vi "Y5140_RdCurr.vi"(8 "error in (no error)":errorcluster caption="错误输入（无错误）", 11 "MyIndex":u8) -> (0 "error out":errorcluster caption="错误输出", 1 "T/F":bool, 2 "Value":sgl)   [LabVIEW 2015]
uses:
  <vilib>/Instr/_visa.llb/VISA Configure Serial Port (Instr).vi
panel:
  out "VISA":refnum<visa-resource-name> caption="VISA资源名称输出"
  out "Rx":string
  out "Tx":string
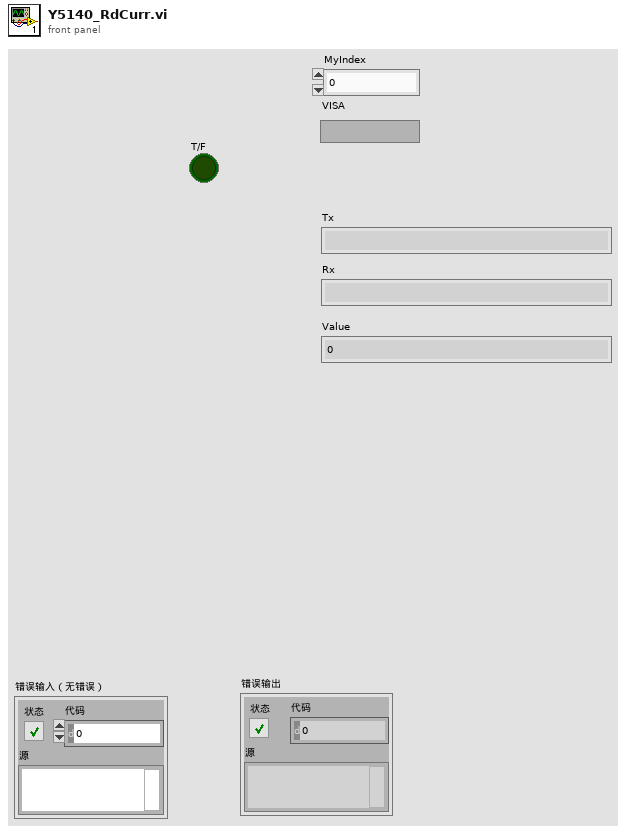
[diagram p1: front panel]
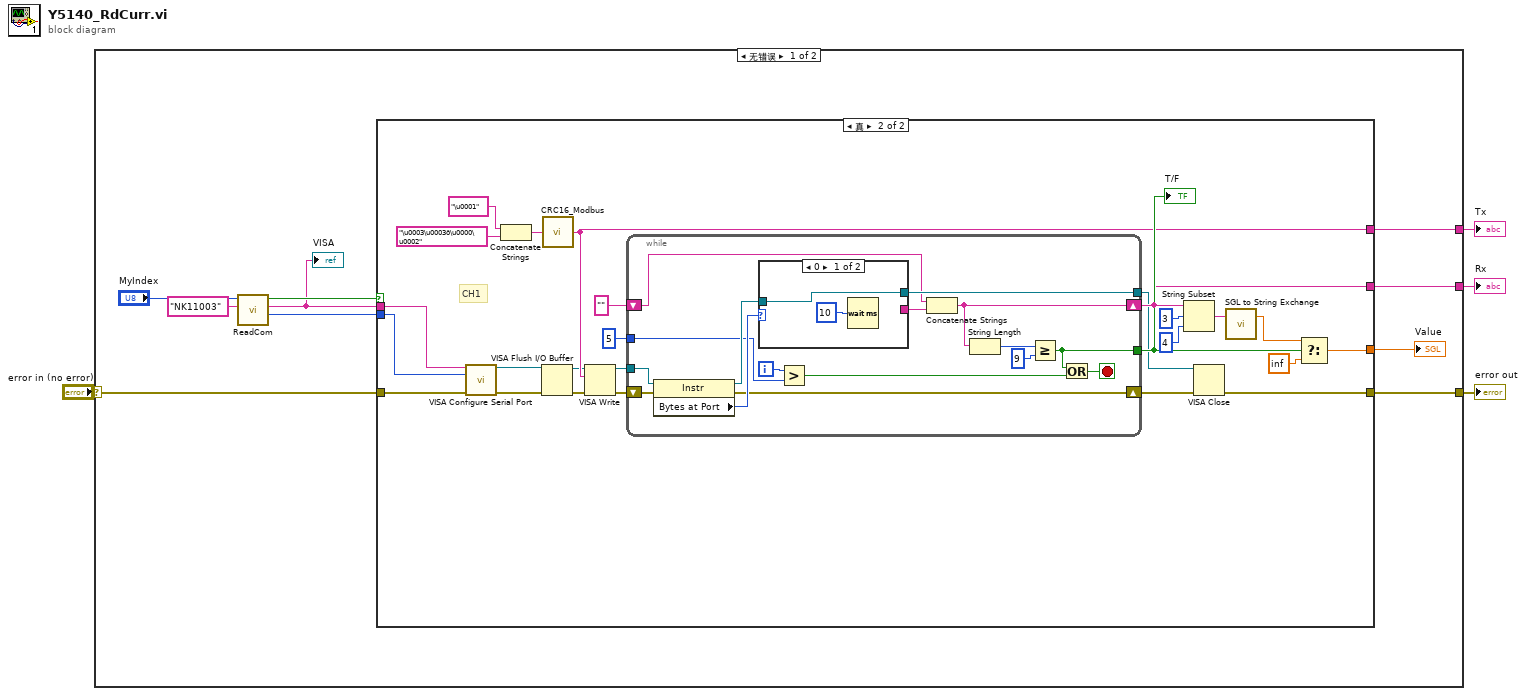
[diagram p0: block diagram]
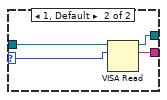
[diagram p3: hidden frame]
diagram:
  n1 = case shown="无错误" "error in (no error)" {
    selector: "error in (no error)" -> [w13 w63]
    tunnel: [w12 w63] -> w3
    tunnel: [w11 _] -> w2
    tunnel: [w10 _] -> w1
    frame No Error {
      n2 = call "ReadCom.vi"("仪器名称"="NK11003", "MyIndex"="MyIndex") -> ("Baudrate"=w5:i32, "COM"=w6:string, "OK?"=w7:bool)  [unwired: 7 in]
      "VISA" <- w6
      n3 = case shown="真" w7 {
        tunnel: [_ w39] -> w14
        tunnel: w13 -> [_ w38]
        tunnel: [_ w16] -> w12
        tunnel: [_ w36] -> w11
        tunnel: [_ w35] -> w10
        tunnel: w6 -> [_ w18]
        tunnel: w5 -> [_ w19]
        frame False {
        }
        frame True {
          # "CH1"
          n4 = call-poly "VISA Configure Serial Port"("VISA resource name"=w18, "baud rate (9600)"=w19, "error in (no error)"=w38) -> ("VISA resource name out"=w17:refnum<visa-resource-name>, "error out"=w20:errorcluster)  [unwired: 11 in]
          n5 = Concatenate Strings("\u0001", "\u0003\u0003ð\u0000\u0002") -> (w22:string)
          n6 = VISA Flush I/O Buffer(VISA resource name=w17, error in (no error)=w20) -> (VISA resource name out=w34:refnum<visa-resource-name>, error out=w33:errorcluster)  [unwired: 1 in]
          n7 = call "CRC16_Modbus.vi"("需要校验的数据"=w22) -> ("String+CRC16"=w36:string)
          n8 = VISA Write(VISA resource name=w34, write buffer=w36, error in (no error)=w33) -> (VISA resource name out=w32:refnum<visa-resource-name>, error out=w31:errorcluster)  [unwired: 1 out]
          n9 = while {
            tunnel: w32 -> [w56]
            tunnel: [w53] -> w15
            shift-right: [w45] -> w35
            shift-left: "" -> [w51]
            tunnel: 5 ("y") -> [w49]
            tunnel: [w41] -> w40
            shift-right: [w47] -> w37
            shift-left: w31 -> [w48]
            i -> [w50]
            stop <- w42 stop-if-true
            n10 = property class="Instr"(reference=w56, error in=w48) -> (reference out=w54:refnum<visa-resource-name>, error out=w47:errorcluster, "Bytes at Port"=w55:u32)
            n11 = case shown="0" w55 {
              selector: w55 -> [_ w61]
              tunnel: w54 -> [w58 w62]
              tunnel: [w58 w60] -> w53
              tunnel: [_ w59] -> w52
              frame 0 {
                n12 = Wait (ms)(milliseconds to wait=u32 10 ("等待时间（毫秒）")) -> ()  [unwired: 1 out]
              }
              frame 1, Default {
                n13 = VISA Read(VISA resource name=w62, byte count=w61) -> (VISA resource name out=w60:refnum<visa-resource-name>, read buffer=w59:string)  [unwired: 1 in, 2 out]
              }
            }
            n14 = Greater?(x=w50, y=w49) -> (0:w46:bool)
            n15 = Concatenate Strings(w51, w52) -> (w45:string)
            n16 = String Length(string=w45) -> (length=w44:i32)
            n17 = Greater Or Equal?(x=w44, y=9) -> (x >= y?=w41:bool)
            n18 = Or(x=w41, y=w46) -> (x .or. y?=w42:bool)
          }
          "T/F" <- w40
          n19 = String Subset(string=w35, offset (0)=3 ("偏移量(0)"), length (rest)=4 ("长度（剩余）")) -> (substring=w26:string)
          n20 = VISA Close(VISA resource name=w15, error in (no error)=w37) -> (error out=w16:errorcluster)
          n21 = call "SGL to String Exchange.vi"("4字节字符串"=w26) -> ("IEE754Floatout"=w25:sgl)  [unwired: 1 in, 1 out]
          n22 = Select(t=w25, s=w40, f=sgl inf) -> (s? t:f=w39:sgl)
        }
      }
      "Value" <- w14
    }
    frame Error {
    }
  }
  "error out" <- w3
  "Tx" <- w2
  "Rx" <- w1
